vi "image file extension.vi"(11 "File Type":T1) -> (3 "Extension":string)   [LabVIEW 2012, in "Camera SubVIs.lvlib"]
uses:
  Camera SubVIs.lvlib
  Image File Type.ctl
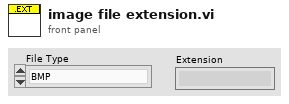
[diagram p1: front panel]
types:
  T1 = typedef "Camera SubVIs.lvlib/Image File Type.ctl" = enum16{"BMP", "JPEG", "JPEG 2000", "PNG", "PNG with Vision Info", "TIFF"}
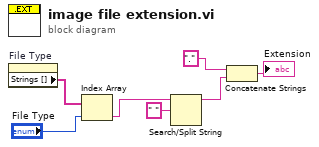
[diagram p0: block diagram]
diagram:
  n1 = property on="File Type" class="Enum (strict)"() -> ("Strings []"=w7:string[])  [unwired: 2 in, 2 out]
  n2 = Index Array(array=w7, index="File Type") -> (element=w5:string)
  n3 = Search/Split String(string=w5, search string/char (-)=" ") -> (substring before match=w2:string)  [unwired: 1 in, 2 out]
  n4 = Concatenate Strings(".", w2) -> (→"Extension":string)
